vi "auto powert supply.vi"() -> ()   [LabVIEW 2017]
uses:
  <instrlib>/Keysight E36300 Series/Keysight E36300 Series.lvlib
panel:
  in  "Channel (1) 2":string="1"
  in  "VISA resource name 3":refnum<visa-resource-name>
  out "?":dbl[](array[numeric]) format="%.3g"
  out "?":dbl[](array[numeric]) format="%.3g"
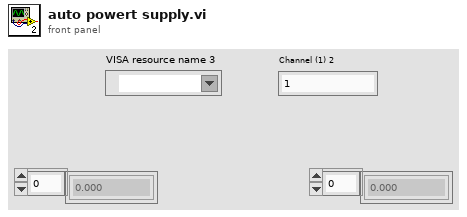
[diagram p1: front panel]
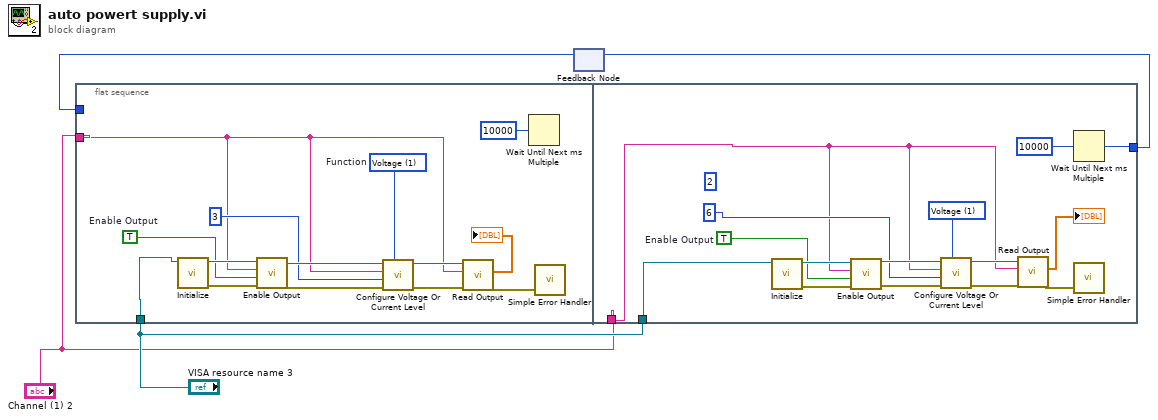
[diagram p0: block diagram]
diagram:
  n1 = flat-sequence {
    tunnel: w2 -> [_]
    tunnel: "VISA resource name 3" -> [w10]
    tunnel: "Channel (1) 2" -> [w7]
    tunnel: [w32] -> w4
    tunnel: "VISA resource name 3" -> [w23]
    tunnel: "Channel (1) 2" -> [w20]
    frame #0 {
      w13 = 1 items=["Current", "Voltage"]  # Function
      w6 = TRUE  # Enable Output
      n2 = call <instrlib>:"Initialize.vi"("VISA resource name"=w10) -> ("error out"=w16:errorcluster, "VISA resource name out"=w17:refnum<visa-resource-name>)  [unwired: 9 in]
      n3 = call <instrlib>:"Enable Output.vi"("error in (no error)"=w16, "Enable Output (F: Disable)"=w6, "Channel (1)"=w7, "VISA resource name"=w17) -> ("error out"=w14:errorcluster, "VISA resource name out"=w15:refnum<visa-resource-name>)  [unwired: 6 in]
      n4 = call <instrlib>:"Configure Voltage Or Current Level.vi"("Function (0 : Current)"=w13, "error in (no error)"=w14, "Voltage Or Current Level (1)"=u32 3 ("millisecond multiple"), "Channel (1)"=w7, "VISA resource name"=w15) -> ("error out"=w8:errorcluster, "VISA resource name out"=w9:refnum<visa-resource-name>)  [unwired: 5 in]
      n5 = call <instrlib>:"Read Output.vi"("error in (no error)"=w8, "Channel (1)"=w7, "VISA resource name"=w9) -> ("error out"=w12:errorcluster, "Actual Voltage Level (V)"=→"?":dbl[])  [unwired: 5 in, 2 out]
      n6 = Wait Until Next ms Multiple(millisecond multiple=u32 10000) -> ()  [unwired: 1 out]
      n7 = call <vilib>:"Simple Error Handler.vi"("error in (no error)"=w12) -> ()  [unwired: 4 in, 5 out]
    }
    frame #1 {
      (unwired) u32 2 ("millisecond multiple")
      w26 = 1 items=["Current", "Voltage"]
      w28 = TRUE  # Enable Output
      n8 = call <instrlib>:"Initialize.vi"("VISA resource name"=w23) -> ("error out"=w30:errorcluster, "VISA resource name out"=w31:refnum<visa-resource-name>)  [unwired: 9 in]
      n9 = call <instrlib>:"Enable Output.vi"("error in (no error)"=w30, "Enable Output (F: Disable)"=w28, "Channel (1)"=w20, "VISA resource name"=w31) -> ("error out"=w27:errorcluster, "VISA resource name out"=w29:refnum<visa-resource-name>)  [unwired: 6 in]
      n10 = call <instrlib>:"Configure Voltage Or Current Level.vi"("Function (0 : Current)"=w26, "error in (no error)"=w27, "Voltage Or Current Level (1)"=u32 6 ("millisecond multiple"), "Channel (1)"=w20, "VISA resource name"=w29) -> ("error out"=w21:errorcluster, "VISA resource name out"=w22:refnum<visa-resource-name>)  [unwired: 5 in]
      n11 = call <instrlib>:"Read Output.vi"("error in (no error)"=w21, "Channel (1)"=w20, "VISA resource name"=w22) -> ("error out"=w25:errorcluster, "Actual Voltage Level (V)"=→"?":dbl[])  [unwired: 5 in, 2 out]
      n12 = Wait Until Next ms Multiple(millisecond multiple=u32 10000) -> (millisecond timer value=w32:u32)
      n13 = call <vilib>:"Simple Error Handler.vi"("error in (no error)"=w25) -> ()  [unwired: 4 in, 5 out]
    }
  }
  n14 = feedback-in #1(w4) -> ()
  n15 = feedback #1() -> (w2:u32)  [unwired: 1 in]
